vi "Set path.vi"(8 "error in (no error)":errorcluster, 10 "path":path, 11 "system object in":refnum<class "system object.lvclass">) -> (0 "error out":errorcluster, 3 "system object out":refnum<class "system object.lvclass">)   [LabVIEW 2020, in "system object.lvclass"]
uses:
  system object.lvclass
  system object.lvclass/system object.ctl
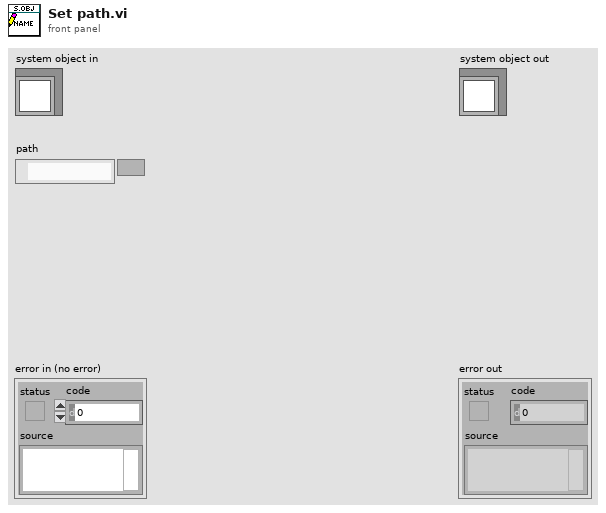
[diagram p1: front panel]
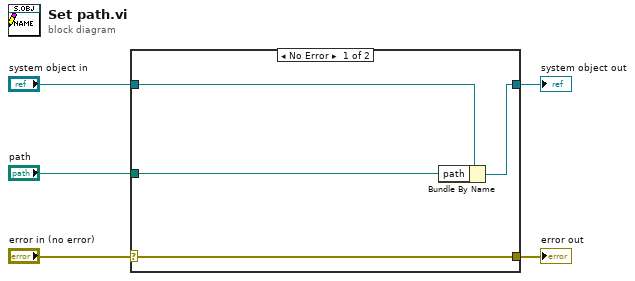
[diagram p0: block diagram]
diagram:
  n1 = case shown="No Error" "error in (no error)" {
    selector: "error in (no error)" -> [w9 w10]
    tunnel: [w9 w10] -> w4
    tunnel: [w7 w11] -> w2
    tunnel: "system object in" -> [w8 w11]
    tunnel: "path" -> [w6 _]
    frame No Error {
      n2 = Bundle By Name(cluster=w8, "path"=w6) -> (w7:refnum<class "system object.lvclass">)
    }
    frame Error {
    }
  }
  "error out" <- w4
  "system object out" <- w2
